vi "PCO_SetPowerSaveMode.vi"(8 "error in (no error)":errorcluster {"code" format="%x"}, 9 "wDelayMinutes":u16, 10 "wMode":u16(ring) items=["OFF", "ON"], 11 "ph":u64) -> (0 "error out":errorcluster {"code" format="%x"}, 2 "ErrorMessage":i32 format="%x", 3 "ph out":u64)   [LabVIEW 2020, in "SDK.lvlib" / "SpecialCommandsDimax.lvlib"]
doc: "<b>Description:</b>\nThis function does set the power save mode of the camera.\n\n<b>Supported camera type:</b>\npco.dimax\n\n<b>Descriptor dependency:</b>\nwPowerDownModeDESC"
uses:
  SpecialCommandsDimax.lvlib
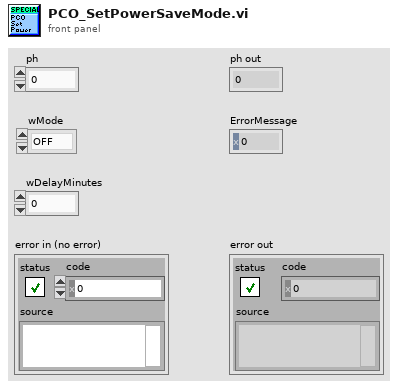
[diagram p1: front panel]
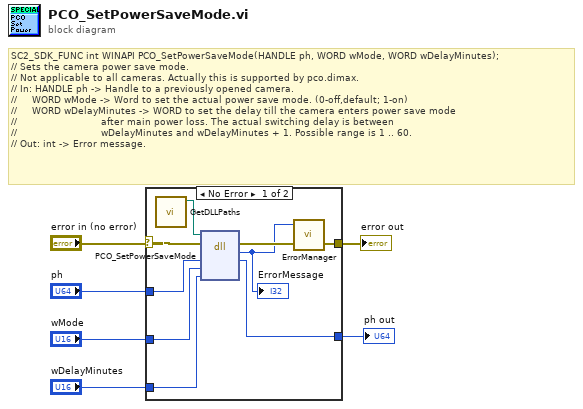
[diagram p0: block diagram]
diagram:
  # "SC2_SDK_FUNC int WINAPI PCO_SetPowerSaveMode(HANDLE ph, WORD wMode, WORD wDelayMinutes);\n// Sets the camera power save mode.\n// Not applicable to all cameras. Actually this is supported by pco.dimax.\n// In: HANDLE ph -> Handle to a previously opened camera.\n//     WORD wMode -> Word to set the actual power save mode. (0-off,default; 1-on)\n//     WORD wDelayMinutes -> WORD to set the delay till the camera enters power save mode\n//                            after main power loss. The actual switching delay is between\n//                            wDelayMinutes and wDelayMinutes + 1. Possible range is 1 .. 60.\n// Out: int -> Error message."
  n1 = case shown="No Error" "error in (no error)" {
    selector: "error in (no error)" -> [w11 w17]
    tunnel: "ph" -> [w15 w16]
    tunnel: [w14 w16] -> w5
    tunnel: "wMode" -> [w13 _]
    tunnel: "wDelayMinutes" -> [w12 _]
    tunnel: [w9 w17] -> w2
    frame No Error {
      n2 = call "GetDLLPaths.vi"() -> ("SC2_Cam_Path"=w7:path)  [unwired: 9 in, 2 out]
      n3 = dll-call lib="?" fn="PCO_SetPowerSaveMode"(path in=w7, error in=w11, "ph"=w15, "wMode"=w13, "wDelayMinutes"=w12) -> (error out=w10:errorcluster, "return type"=w8:i32, "ph"=w14:u64)  [unwired: 3 in, 1 out]
      "ErrorMessage" <- w8
      n4 = call "ErrorManager.vi"("error in (no error)"=w10, "error code"=w8) -> ("error out"=w9:errorcluster)  [unwired: 3 in]
    }
    frame Error {
    }
  }
  "ph out" <- w5
  "error out" <- w2
